vi "Returning Values By Reference Array Of Simple Struct Complete.vi"() -> ()   [LabVIEW 2009, in "LabVIEWWrapper_PassingDataSampleDLL.lvlib"]
doc: "void ReturningValuesByReference_ArrayOfSimpleStruct (struct simpleStructCircle **circleArray, int length);"
uses:
  LabVIEWWrapper_PassingDataSampleDLL.lvlib
  CustomControlsForStructs/SimpleStruct Circle.ctl
panel:
  out "Destination":T1[](array[typedef])
  in  "length":i32
  in  "error in (no error)":errorcluster
  out "newLength out":i32
  out "newArray out":i32
  out "error out":errorcluster
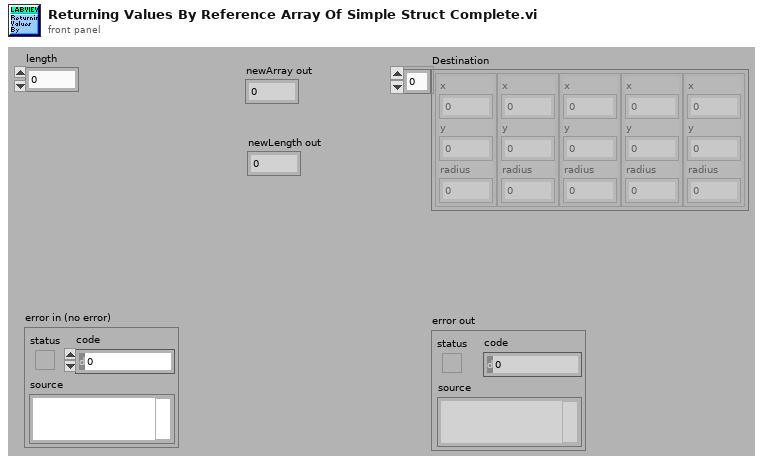
[diagram p1: front panel]
types:
  T1 = typedef "LabVIEWWrapper_PassingDataSampleDLL.lvlib/SimpleStruct Circle.ctl" = cluster{"x":sgl, "y":sgl, "radius":sgl}
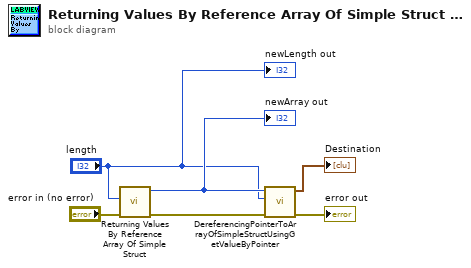
[diagram p0: block diagram]
diagram:
  n1 = call "Returning Values By Reference Array Of Simple Struct.vi"("error in (no error)"="error in (no error)", "length"="length") -> ("error out"=w5:errorcluster, "circleArray out"=w2:i32)  [unwired: 8 in]
  "newArray out" <- w2
  n2 = call "DereferencingPointerToArrayOfSimpleStructUsingGetValueByPointer.vi"("error in (no error)"=w5, "Length"="length", "Address (Pointer)"=w2) -> ("error out"=→"error out":errorcluster, "Destination"=→"Destination":T1[])  [unwired: 7 in]
  "newLength out" <- "length"
